vi "Simple_Lag_Filter.vi"(10 "Input":dbl, 11 "Lag":dbl min=0.0 max=1.0) -> (3 "Lagged Ouptut":dbl)   [LabVIEW 2019]
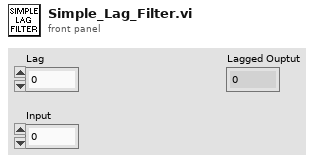
[diagram p1: front panel]
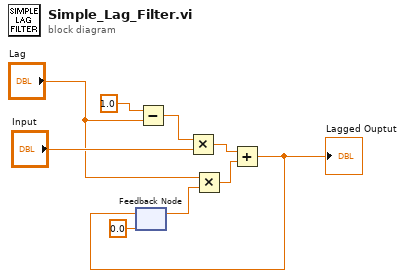
[diagram p0: block diagram]
diagram:
  n1 = feedback #1(0.0 ("Normalized Left Wheel Demand")) -> (w6:dbl)
  n2 = Subtract(x=1.0, y="Lag") -> (x-y=w2:dbl)
  n3 = Multiply(x=w2, y="Input") -> (x*y=w8:dbl)
  n4 = Multiply(x="Lag", y=w6) -> (x*y=w9:dbl)
  n5 = Add(x=w8, y=w9) -> (x+y=w3:dbl)
  "Lagged Ouptut" <- w3
  n6 = feedback-in #1(w3) -> ()
